vi "setTimebase.vi"(8 "error in (no error)":errorcluster, 9 "Delay [s]":dbl, 10 "Timebase [s/Div]":dbl, 11 "ScopeNi in":refnum<class "ScopeNi.lvclass">) -> (0 "error out":errorcluster, 3 "ScopeNi out":refnum<class "ScopeNi.lvclass">)   [LabVIEW 2023, in "ScopeNi.lvclass"]
doc: "<b>Author:</b> Wolfgang\n<b>Description:</b> Configure the timebase"
uses:
  ScopeNi.lvclass
  ScopeNi.lvclass/ScopeNi.ctl
panel:
  in  "samples/second":dbl=100000000.0 format="%#_13p"
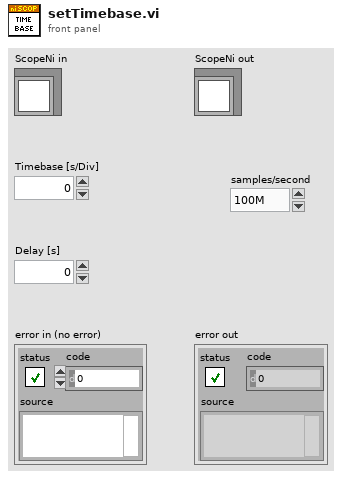
[diagram p1: front panel]
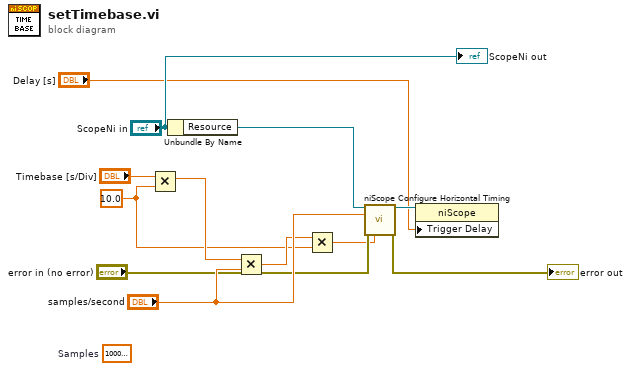
[diagram p0: block diagram]
diagram:
  (unwired) 10000000.0  # Samples
  w1 = 10.0 ("y")
  n1 = Multiply(x="Timebase [s/Div]", y=w1) -> (x*y=w5:dbl)
  n2 = Unbundle By Name("ScopeNi in") -> ("Resource"=w11:refnum<k15>)
  n3 = Multiply(x=w5, y="samples/second") -> (x*y=w9:dbl)
  n4 = Multiply(x=w9, y=w1) -> (x*y=w2:dbl)
  n5 = call <instrlib>:"niScope Configure Horizontal Timing.vi"("instrument handle"=w11, "min sample rate"="samples/second", "error in"="error in (no error)", "min record length"=w2) -> ("instrument handle out"=w4:refnum<k15>, "error out"=→"error out":errorcluster)  [unwired: 10 in]
  n6 = property class="niScope"(reference=w4, "Trigger Delay"="Delay [s]") -> ()  [unwired: 1 in, 2 out]
  "ScopeNi out" <- "ScopeNi in"
